vi "zeroAndSpan.vi"(5 "usefulMax":dbl, 7 "usefulMin":dbl, 8 "spanValue":dbl, 9 "zeroValue":dbl, 10 "DesiredValue":dbl=nan, 11 "MeasuredPercent":dbl) -> (1 "Message":string, 2 "PercentToSet":dbl, 3 "calibratedOutput":dbl)   [LabVIEW 2016]
doc: "Takes Percent-of-range data and applies calibration in the form of Zero and Span readings\nOr takes desired value, and computes percent of range"
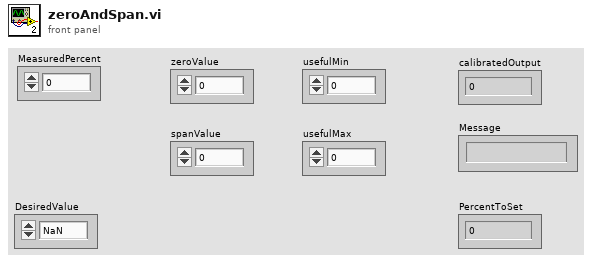
[diagram p1: front panel]
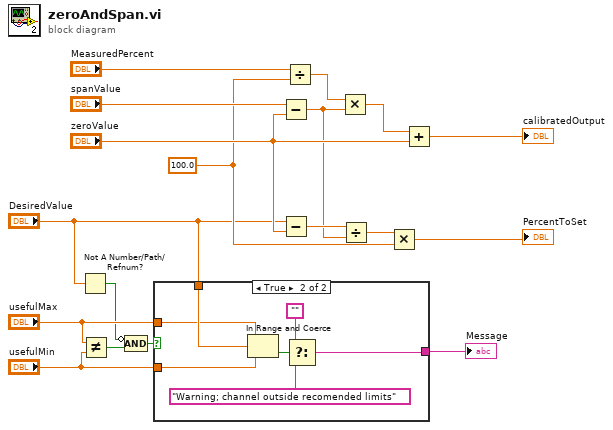
[diagram p0: block diagram]
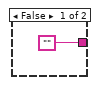
[diagram p2: hidden frame]
diagram:
  w5 = 100.0 ("y")
  n1 = Not A Number/Path/Refnum?(number/path/refnum="DesiredValue") -> (NaN/Path/Refnum?=w2:bool)
  n2 = Not Equal?(x="usefulMax", y="usefulMin") -> (x != y?=w3:bool)
  n3 = Compound Arithmetic op=AND(invert w2, w3) -> (w4:bool)
  n4 = case shown="True" w4 {
    tunnel: ["" w25] -> w18
    tunnel: "DesiredValue" -> [_ w22]
    tunnel: "usefulMax" -> [_ w21]
    tunnel: "usefulMin" -> [_ w20]
    frame False {
    }
    frame True {
      n5 = In Range and Coerce(upper limit=w21, x=w22, lower limit=w20) -> (In Range?=w23:bool)  [unwired: 1 out]
      n6 = Select(t="", s=w23, f="Warning; channel outside recomended limits") -> (s? t:f=w25:string)
    }
  }
  "Message" <- w18
  n7 = Subtract(x="spanValue", y="zeroValue") -> (x-y=w8:dbl)
  n8 = Subtract(x="DesiredValue", y="zeroValue") -> (x-y=w9:dbl)
  n9 = Divide(x="MeasuredPercent", y=w5) -> (x/y=w15:dbl)
  n10 = Multiply(x=w15, y=w8) -> (x*y=w14:dbl)
  n11 = Divide(x=w9, y=w8) -> (x/y=w7:dbl)
  n12 = Multiply(x=w7, y=w5) -> (x*y=→"PercentToSet":dbl)
  n13 = Add(x=w14, y="zeroValue") -> (x+y=→"calibratedOutput":dbl)
